vi "Main.vi"(11 "Module Admin":refnum<class "Delacor_lib_QMH_Module Admin.lvclass">) -> ()   [LabVIEW 2020, in "FileLogging.lvlib"]
doc: "This template is based off of the Queued Message Handler design pattern and the Queued Message Handler project template that ships with LabVIEW.\n\nThe main difference is that the queue is private to this module and communication between modules is performed via Broadcast and Request events.\n\nRequest events are wrapped in public API methods and are handled in the Event Handling Loop (EHL) of this VI. Any module can register for Broadcast events sent by this module. The EHL generates messages based on user interface actions.\n\nThe Message Handling Loop (MHL) processes messages generated by the EHL, or by other messages. The messages are string values, so new messages can be added easily to the Message Cases case structure in the MHL. Each message cluster can also provide an optional value for Message Data, which is a variant that can be converted to whatever message-specific data is required.\n_____\nBased on Delacor QMH Project Template 4.0.0.47.\n_____\nBased on Delacor QMH Project Template 5.0.0.82."
uses:
  FileLogging.lvlib
  <vilib>/Delacor/Delacor QMH/Libraries/Module Admin_class/Delacor_lib_QMH_Module Admin.lvclass
  Module Data--cluster.ctl
  Stop Argument--cluster.ctl
  <vilib>/Delacor/Delacor QMH/Libraries/Message Queue_class/Delacor_lib_QMH_Message Queue.lvclass/Delacor_lib_QMH_Message Queue.ctl
  <vilib>/Delacor/Delacor QMH/Libraries/Module Admin_class/Delacor_lib_QMH_Module Admin.lvclass/Delacor_lib_QMH_Module Admin.ctl
  Initialize File Argument--cluster.ctl
  Initialize File (Reply Payload)--cluster.ctl
  Log Data Argument--cluster.ctl
  Stop Logging Argument--cluster.ctl
  Settings Editor/Update Application Settings (Reply Payload)--cluster.ctl
  Settings Editor/Settings--cluster.ctl
  <vilib>/Utility/miscctls.llb/LVPointTypeDef.ctl
  <vilib>/Delacor/Delacor QMH/Libraries/Message Queue_class/Delacor_lib_QMH_Enqueue Message (Single).vi
  <vilib>/Delacor/Delacor QMH/Libraries/Module Admin_class/Delacor_lib_QMH_Get External Launch.vi
  <vilib>/Utility/error.llb/Error Cluster From Error Code.vi
  <vilib>/ErrorRing/Error Ring.xnode
  <vilib>/Delacor/Delacor QMH/Libraries/Message Queue_class/Delacor_lib_QMH_Message Queue.lvclass
  Settings Editor/Settings Editor.lvlib
panel:
  out "Settings":T1
  out "error out":errorcluster
  # "This is a headless module. Show its panel to confirm that the Settings are updated correctly and other debugging tasks. Use the Settings Editor to change the settings for this module."
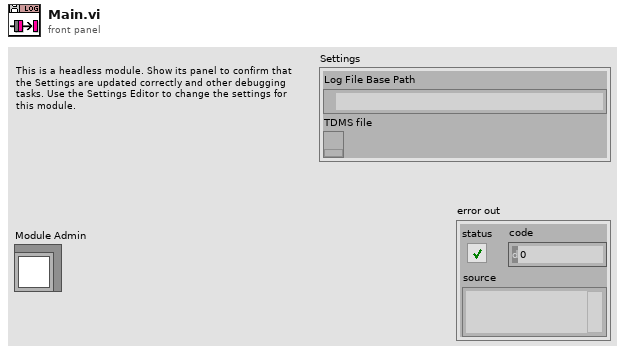
[diagram p1: front panel]
types:
  T1 = typedef "FileLogging.lvlib/Module Data--cluster.ctl" = cluster{"Log File Base Path":path, "TDMS file":refnum<k34>}
  T2 = typedef "Settings Editor.lvlib/Broadcast Events--cluster.ctl" = cluster{"Module Did Init":refnum<user-event>, "Status Updated":refnum<user-event>, "Error Reported":refnum<user-event>, "Module Did Stop":refnum<user-event>, "Update Module Execution Status":refnum<user-event>, "Application Settings Updated":refnum<user-event>}
  T3 = typedef "FileLogging.lvlib/Request Events--cluster.ctl" = cluster{"Stop Module":refnum<user-event>, "Show Panel":refnum<user-event>, "Hide Panel":refnum<user-event>, "Get Module Execution Status":refnum<user-event>, "Show Diagram":refnum<user-event>, "Stop Logging":refnum<user-event>, "Log Data":refnum<user-event>, "Initialize File":refnum<user-event>}
  T4 = enum32{"invalid lock state", "Not Locked", "Locked (No Password)", "Password-protected"}
  T5 = typedef "FileLogging.lvlib/Stop Argument--cluster.ctl" = cluster{"Origin":string, "Exit via Stop Module Req?":bool, "Wait for Module to stop?":bool}
  T6 = typedef "FileLogging.lvlib/Initialize File Argument--cluster.ctl" = cluster{"Wait Notifier":refnum<notifier>, "wait for reply":bool}
  T7 = typedef "FileLogging.lvlib/Log Data Argument--cluster.ctl" = cluster{"Waveforms":waveform(dbl)[]}
  T8 = typedef "FileLogging.lvlib/Stop Logging Argument--cluster.ctl" = cluster{"Boolean":bool}
  T9 = typedef "Settings Editor.lvlib/Update Application Settings (Reply Payload)--cluster.ctl" = cluster{"Settings":T10, "Update Settings_error":errorcluster}
  T10 = typedef "Settings Editor.lvlib/Settings--cluster.ctl" = cluster{"Log File Base Path":path, "Analog Input Channel":refnum<k21>, "Units":i32}
  T11 = typedef "LVPointTypeDef.ctl" = cluster{"Horizontal":i16, "Vertical":i16}
  T12 = enum32{"Invalid", "Standard", "Closed", "Hidden", "Minimized", "Maximized"}
  T13 = typedef "FileLogging.lvlib/Initialize File (Reply Payload)--cluster.ctl" = cluster{"File Path":path, "Initialize File_error":errorcluster}
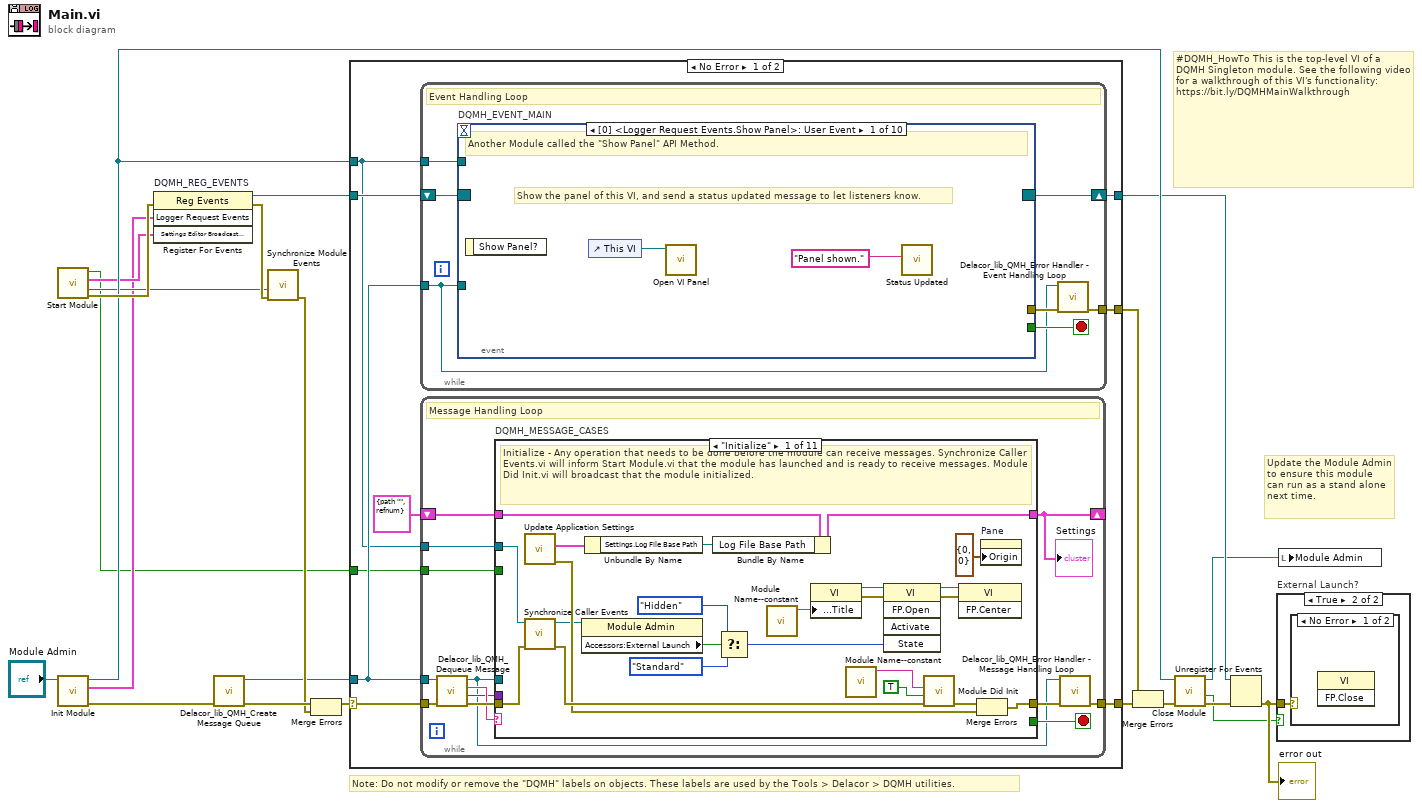
[diagram p0: block diagram]
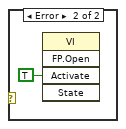
[diagram p3: hidden frame]
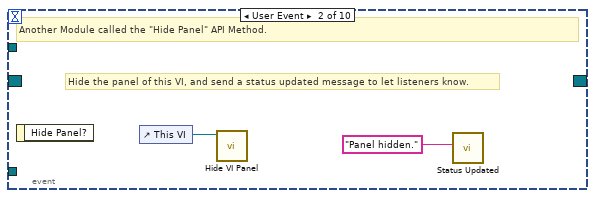
[diagram p4: hidden frame]
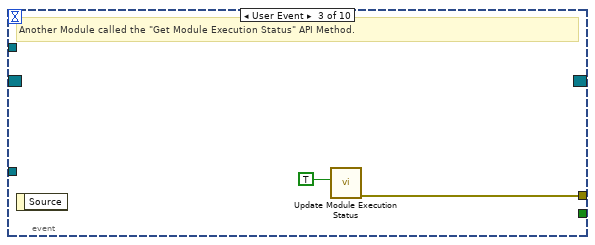
[diagram p5: hidden frame]
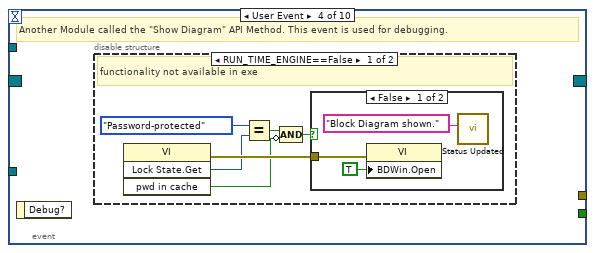
[diagram p6: hidden frame]
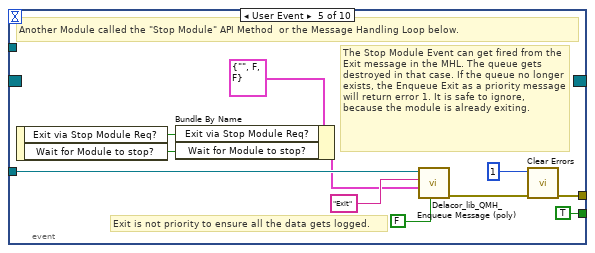
[diagram p9: hidden frame]
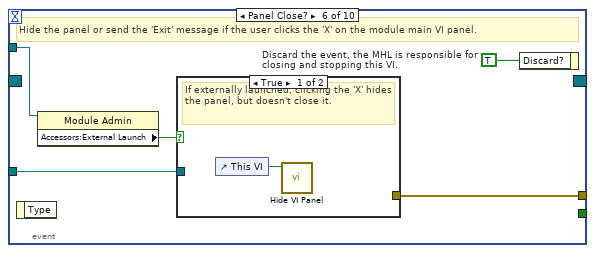
[diagram p10: hidden frame]
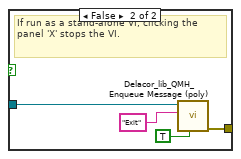
[diagram p11: hidden frame]
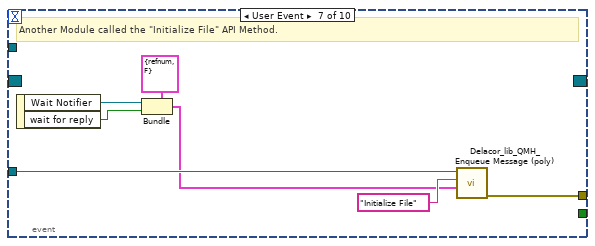
[diagram p12: hidden frame]
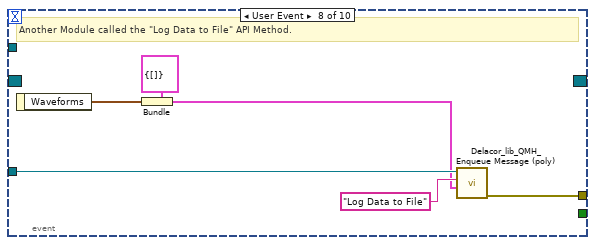
[diagram p13: hidden frame]
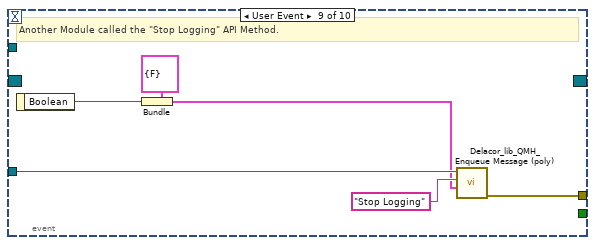
[diagram p14: hidden frame]
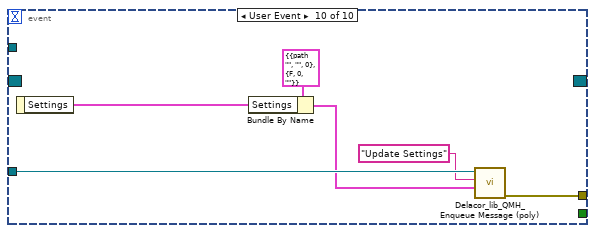
[diagram p15: hidden frame]
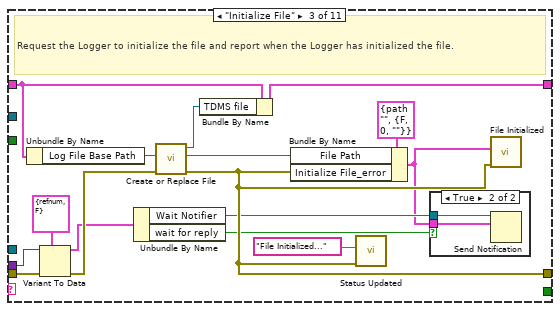
[diagram p17: hidden frame]
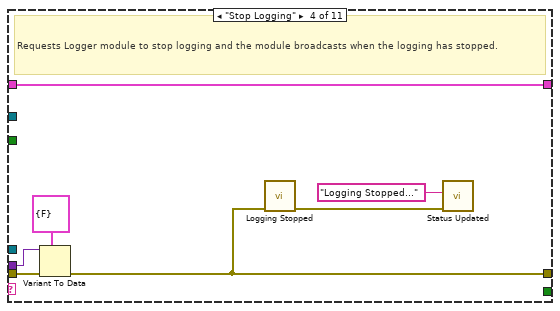
[diagram p19: hidden frame]
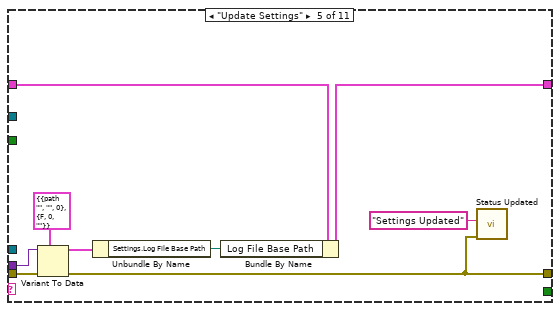
[diagram p20: hidden frame]
diagram:
  # "#DQMH_HowTo This is the top-level VI of a DQMH Singleton module. See the following video for a walkthrough of this VI's functionality: https://bit.ly/DQMHMainWalkthrough"
  # "Note: Do not modify or remove the \"DQMH\" labels on objects. These labels are used by the Tools > Delacor > DQMH utilities."
  # "Update the Module Admin to ensure this module can run as a stand alone next time."
  n1 = call "Start Module.vi"() -> ("error out"=w14:errorcluster, "Wait for Event Sync?"=w4:bool, "Settings Editor Broadcast Events"=w3:T2, "Module Was Already Running?"=w1:bool)  [unwired: 8 in]
  n2 = call "Init Module.vi"("Singleton Module Admin in"="Module Admin") -> ("error out"=w21:errorcluster, "Logger Request Events"=w2:T3, "Singleton Module Admin out"=w11:refnum<class "Delacor_lib_QMH_Module Admin.lvclass">)  [unwired: 8 in]
  n3 = register-events "DQMH_REG_EVENTS"(error in=w14, w2, w3) -> (reference out=w9:refnum<event-registration>, error out=w13:errorcluster)  [unwired: 1 in]
  n4 = call <vilib>:"Delacor_lib_QMH_Create Message Queue.vi"("error in (no error)"=w21) -> ("error out"=w16:errorcluster, "Message Queue"=w8:refnum<class "Delacor_lib_QMH_Message Queue.lvclass">)  [unwired: 9 in]
  n5 = call "Synchronize Module Events.vi"("error in (no error)"=w13, "Wait for Event Sync?"=w4) -> ("error out"=w12:errorcluster)  [unwired: 9 in]
  n6 = Merge Errors(w16, w12) -> (w15:errorcluster)
  n7 = case shown="No Error" w15 {
    selector: w15 -> [w29 w237]
    tunnel: [w31 w236] -> w22
    tunnel: [w28 w244] -> w10
    tunnel: w9 -> [w26 w244]
    tunnel: w8 -> [w25 w238]
    tunnel: [w30 _] -> w19
    tunnel: w11 -> [w24 w240]
    tunnel: w1 -> [w23 w239]
    frame No Error {
      n8 = while {
        tunnel: w25 -> [w32]
        shift-right: [w35] -> w28
        shift-left: w26 -> [w36]
        tunnel: [w37] -> w30
        tunnel: w24 -> [w33]
        stop <- w34 stop-if-true
        # "Event Handling Loop"
        n9 = event "DQMH_EVENT_MAIN" shown="[0] <Logger Request Events.Show Panel>: User Event" {
          selector: w36 -> [_ _ _ _ _ _ _ _ _ _]
          dyn-events: [_ _ _ _ _ _ _ _ _ _] -> w35
          timeout: _ -> [_ _ _ _ _ _ _ _ _ _]
          tunnel: [_ _ _ _ TRUE ("Discard?") _ _ _ _ _] -> w34
          tunnel: w32 -> [_ _ _ _ w60 w67 w80 w86 w92 w98]
          tunnel: [_ _ w44 _ w63 w69 w81 w87 w93 w99] -> w38
          tunnel: w33 -> [_ _ _ _ _ w66 _ _ _ _]
          event User Event {
            # "Show the panel of this VI, and send a status updated message to let listeners know."
            # "Another Module called the \"Show Panel\" API Method."
            n10 = event-data() -> ()  [unwired: 1 in, 1 out]
            n11 = control-ref of="This VI"() -> (w40:refnum<vi>)
            n12 = call "Open VI Panel.vi"("VI"=w40) -> ()  [unwired: 10 in, 1 out]
            n13 = call "Status Updated.vi"("Status"="Panel shown." ("format string")) -> ()  [unwired: 10 in, 1 out]
          }
          event User Event {
            # "Hide the panel of this VI, and send a status updated message to let listeners know."
            # "Another Module called the \"Hide Panel\" API Method."
            n14 = event-data() -> ()  [unwired: 1 in, 1 out]
            n15 = control-ref of="This VI"() -> (w42:refnum<vi>)
            n16 = call "Hide VI Panel.vi"("VI"=w42) -> ()  [unwired: 10 in, 1 out]
            n17 = call "Status Updated.vi"("Status"="Panel hidden." ("format string")) -> ()  [unwired: 10 in, 1 out]
          }
          event User Event {
            # "Another Module called the \"Get Module Execution Status\" API Method."
            n18 = event-data() -> ()  [unwired: 1 in, 1 out]
            n19 = call "Update Module Execution Status.vi"("Running?"=TRUE) -> ("error out"=w44:errorcluster)  [unwired: 10 in]
          }
          event User Event {
            # "Another Module called the \"Show Diagram\" API Method. This event is used for debugging."
            n20 = event-data() -> ()  [unwired: 1 in, 1 out]
            n21 = disable-structure shown="RUN_TIME_ENGINE==False" {
              frame condition #0 (active) {
                # "functionality not available in exe"
                n22 = invoke class="VI" method="Lock State.Get"() -> (error out=w50:errorcluster, "Get Lock State"=w49:T4, "pwd in cache"=w46:bool)  [unwired: 4 in, 1 out]
                n23 = Equal?(x=T4."Password-protected", y=w49) -> (x = y?=w47:bool)
                n24 = Compound Arithmetic op=AND(w47, invert w46) -> (w45:bool)
                n25 = case shown="False" w45 {
                  tunnel: w50 -> [w53 _]
                  frame False {
                    n26 = property class="VI"(error in=w53, "BDWin.Open"=TRUE ("Block Diagram Window:Open")) -> ()  [unwired: 1 in, 2 out]
                    n27 = call "Status Updated.vi"("Status"="Block Diagram shown." ("format string")) -> ()  [unwired: 10 in, 1 out]
                  }
                  frame True {
                    # "Password-protected VI, and the password is not in the cache. Do not show the diagram."
                  }
                }
              }
              frame condition #1 {
              }
            }
          }
          event User Event {
            # "Exit is not priority to ensure all the data gets logged."
            # "The Stop Module Event can get fired from the Exit message in the MHL. The queue gets destroyed in that case. If the queue no longer exists, the Enqueue Exit as a priority message will return error 1. It is safe to ignore, because the module is already exiting."
            # "Another Module called the \"Stop Module\" API Method  or the Message Handling Loop below."
            n28 = event-data() -> ("Exit via Stop Module Req?"=w56:bool, "Wait for Module to stop?"=w55:bool)  [unwired: 1 in]
            n29 = Bundle By Name(cluster=T5 {"Origin"="", "Exit via Stop Module Req?"=FALSE, "Wait for Module to stop?"=FALSE} ("Stop Argument"), "Exit via Stop Module Req?"=w56, "Wait for Module to stop?"=w55) -> (w54:T5)
            n30 = call-poly <vilib>:"Delacor_lib_QMH_Enqueue Message (poly).vi"("Priority Message? (F)"=FALSE, "Message Data"=w54, "Message"="Exit", "Message Queue in"=w60) -> ("error out"=w64:errorcluster)  [unwired: 6 in, 1 out]
            n31 = call <vilib>:"Clear Errors.vi"("error in (no error)"=w64, "specific error code to clear (0: all)"=1) -> ("error out"=w63:errorcluster)  [unwired: 4 in, 1 out]
          }
          event Panel Close? {
            w68 = TRUE  # Discard the event, the MHL is responsible for closing and stopping this VI.
            # "Hide the panel or send the 'Exit' message if the user clicks the 'X' on the module main VI panel."
            n32 = event-data() -> ()  [unwired: 1 in, 1 out]
            n33 = property class="Module Admin"(reference=w66) -> ("Accessors:External Launch"=w65:bool)  [unwired: 1 in, 2 out]
            n34 = case shown="True" w65 {
              tunnel: w67 -> [_ w73]
              tunnel: [_ w74] -> w69
              frame True {
                # "If externally launched, clicking the 'X' hides the panel, but doesn't close it."
                n35 = control-ref of="This VI"() -> (w70:refnum<vi>)
                n36 = call "Hide VI Panel.vi"("VI"=w70) -> ()  [unwired: 10 in, 1 out]
              }
              frame False {
                # "If run as a stand-alone VI, clicking the panel 'X' stops the VI."
                n37 = call-poly <vilib>:"Delacor_lib_QMH_Enqueue Message (poly).vi"("Priority Message? (F)"=TRUE, "Message"="Exit", "Message Queue in"=w73) -> ("error out"=w74:errorcluster)  [unwired: 7 in, 1 out]
              }
            }
            n38 = event-data("Discard?"=w68) -> ()  [unwired: 1 in, 1 out]
          }
          event User Event {
            # "Another Module called the \"Initialize File\" API Method."
            n39 = event-data() -> ("Wait Notifier"=w76:refnum<notifier>, "wait for reply"=w75:bool)  [unwired: 1 in]
            n40 = Bundle(cluster=T6 {"Wait Notifier"=refnum, "wait for reply"=FALSE} ("Initialize File Argument"), "Wait Notifier"=w76, "wait for reply"=w75) -> (w77:T6)
            n41 = call-poly <vilib>:"Delacor_lib_QMH_Enqueue Message (poly).vi"("Message Data"=w77, "Message"="Initialize File", "Message Queue in"=w80) -> ("error out"=w81:errorcluster)  [unwired: 7 in, 1 out]
          }
          event User Event {
            # "Another Module called the \"Log Data to File\" API Method."
            n42 = event-data() -> ("Waveforms"=w82:waveform(dbl)[])  [unwired: 1 in]
            n43 = Bundle(cluster=T7 {"Waveforms"=[]} ("Log Data to File Argument"), "Waveforms"=w82) -> (w83:T7)
            n44 = call-poly <vilib>:"Delacor_lib_QMH_Enqueue Message (poly).vi"("Message Data"=w83, "Message"="Log Data to File", "Message Queue in"=w86) -> ("error out"=w87:errorcluster)  [unwired: 7 in, 1 out]
          }
          event User Event {
            # "Another Module called the \"Stop Logging\" API Method."
            n45 = event-data() -> ("Boolean"=w88:bool)  [unwired: 1 in]
            n46 = Bundle(cluster=T8 {"Boolean"=FALSE} ("Stop Logging Argument"), "Boolean"=w88) -> (w89:T8)
            n47 = call-poly <vilib>:"Delacor_lib_QMH_Enqueue Message (poly).vi"("Message Data"=w89, "Message"="Stop Logging", "Message Queue in"=w92) -> ("error out"=w93:errorcluster)  [unwired: 7 in, 1 out]
          }
          event User Event {
            n48 = event-data() -> ("Settings"=w95:T10)  [unwired: 1 in]
            n49 = Bundle By Name(cluster=T9 {"Settings"={"Log File Base Path"=path "", "Analog Input Channel"="", "Units"=0}, "Update Settings_error"={"status"=FALSE, "code"=0, "source"=""}} ("Settings Updated Argument"), "Settings"=w95) -> (w94:T9)
            n50 = call-poly <vilib>:"Delacor_lib_QMH_Enqueue Message (poly).vi"("Message Data"=w94, "Message"="Update Settings", "Message Queue in"=w98) -> ("error out"=w99:errorcluster)  [unwired: 7 in, 1 out]
          }
        }
        n51 = call-dynamic "Delacor_lib_QMH_Error Handler - Event Handling Loop.vi"("error in (no error)"=w38, "Message Queue in"=w32) -> ("dup error in"=w37:errorcluster)  [unwired: 8 in, 1 out]
      }
      n52 = while {
        tunnel: w25 -> [w103]
        shift-right: [w107] -> _
        shift-left: T1 {"Log File Base Path"=path "", "TDMS file"=refnum} ("Data Cluster") -> [w108]
        tunnel: w29 -> [w111]
        tunnel: [w109] -> w31
        tunnel: w24 -> [w101]
        tunnel: w23 -> [w100]
        stop <- w106 stop-if-true
        # "Message Handling Loop"
        n53 = call-dynamic "Delacor_lib_QMH_Dequeue Message.vi"("error in (no error)"=w111, "Message Queue in"=w103) -> ("error out"=w110:errorcluster, "Message Data"=w104:variant, "Message"=w105:string, "Message Queue out"=w102:refnum<class "Delacor_lib_QMH_Message Queue.lvclass">)  [unwired: 6 in]
        n54 = case "DQMH_MESSAGE_CASES" shown="\"Initialize\"" w105 {
          selector: w105 -> [_ _ _ _ _ _ _ _ _ _ w223]
          tunnel: w102 -> [_ _ _ _ _ _ _ _ w189 w213 _]
          tunnel: w110 -> [w133 w137 w152 w162 w171 w180 w183 w185 w196 w219 w225]
          tunnel: [w130 w137 w153 w161 w164 w178 w182 w185 w192 w216 w226] -> w112
          tunnel: w108 -> [w120 w136 w141 w157 w170 w173 w181 w184 w191 w205 w224]
          tunnel: [w114 w136 w140 w157 w168 w173 w181 w184 w191 w205 w224] -> w107
          tunnel: [_ _ _ _ _ _ _ _ _ w212 _] -> w106
          tunnel: w104 -> [_ _ w150 w159 w169 w177 _ _ w190 w211 _]
          tunnel: w101 -> [w121 _ _ _ _ _ _ _ w188 w206 _]
          tunnel: w100 -> [_ _ _ _ _ _ _ _ _ w203 _]
          frame "Initialize" {
            # "Initialize - Any operation that needs to be done before the module can receive messages. Synchronize Caller Events.vi will inform Start Module.vi that the module has launched and is ready to receive messages. Module Did Init.vi will broadcast that the module initialized."
            n55 = call "Update Application Settings.vi"() -> ("error out"=w129:errorcluster, "Reply Payload"=w115:T9)  [unwired: 9 in, 1 out]
            n56 = call "Synchronize Caller Events.vi"("error in (no error)"=w133, "Singleton Module Admin in"=w121) -> ("error out"=w132:errorcluster, "Singleton Module Admin out"=w117:refnum<class "Delacor_lib_QMH_Module Admin.lvclass">)  [unwired: 8 in]
            n57 = property class="Module Admin"(reference=w117) -> ("Accessors:External Launch"=w125:bool)  [unwired: 1 in, 2 out]
            n58 = Unbundle By Name(w115) -> ("Settings.Log File Base Path"=w113:path)
            n59 = Bundle By Name(cluster=w120, "Log File Base Path"=w113) -> (w114:T1)
            n60 = Select(t=T12."Hidden" ("State"), s=w125, f=T12."Standard" ("State")) -> (s? t:f=w122:T12)
            n61 = call "Module Name--constant.vi"() -> ("Module Name"=w128:string)  [unwired: 11 in]
            n62 = property class="VI"("Front Panel.Title"=w128) -> (reference out=w127:refnum<vi>, error out=w135:errorcluster)  [unwired: 2 in]
            n63 = call "Module Name--constant.vi"() -> ("Module Name"=w118:string)  [unwired: 11 in]
            n64 = invoke class="VI" method="FP.Open"(reference=w127, error in=w135, "State"=w122) -> (reference out=w126:refnum<vi>, error out=w134:errorcluster)  [unwired: 2 in, 3 out]
            n65 = call "Module Did Init.vi"("error in (no error)"=w132, "Initialized?"=TRUE, "Origin"=w118) -> ("error out"=w131:errorcluster)  [unwired: 8 in]
            n66 = invoke class="VI" method="FP.Center"(reference=w126, error in=w134) -> ()  [unwired: 1 in, 3 out]
            n67 = Merge Errors(w131, w129) -> (w130:errorcluster)
            n68 = property on="Pane" class="Pane"("Origin"=T11 {"Horizontal"=0, "Vertical"=0}) -> ()  [unwired: 2 in, 2 out]
          }
          frame "--- Module Specific ---" {
            # "Separator -- The following cases handle messages specific to this Module."
          }
          frame "Initialize File" {
            # "Request the Logger to initialize the file and report when the Logger has initialized the file."
            n69 = Unbundle By Name(w141) -> ("Log File Base Path"=w143:path)
            n70 = Variant To Data(error in=w152, type=T6 {"Wait Notifier"=refnum, "wait for reply"=FALSE} ("Initialize File Argument"), Variant=w150) -> (data=w148:T6, error out=w151:errorcluster)
            n71 = Unbundle By Name(w148) -> ("Wait Notifier"=w147:refnum<notifier>, "wait for reply"=w146:bool)
            n72 = call "Create or Replace File.vi"("error in (no error)"=w151, "Log File Base Path"=w143) -> ("error out"=w153:errorcluster, "File Path"=w139:path, "Refnum out"=w142:refnum<k34>)  [unwired: 7 in]
            n73 = Bundle By Name(cluster=w141, "TDMS file"=w142) -> (w140:T1)
            n74 = Bundle By Name(cluster=T13 {"File Path"=path "", "Initialize File_error"={"status"=FALSE, "code"=0, "source"=""}} ("Initialize File (Reply Payload)"), "File Path"=w139, "Initialize File_error"=w153) -> (w144:T13)
            n75 = call "Status Updated.vi"("error in (no error)"=w153, "Status"="File Initialized...") -> ()  [unwired: 9 in, 1 out]
            n76 = case shown="True" w146 {
              tunnel: w147 -> [_ w155]
              tunnel: w144 -> [_ w154]
              frame False {
              }
              frame True {
                n77 = Send Notification(notification=w154, notifier=w155) -> ()  [unwired: 1 in, 2 out]
              }
            }
            n78 = call "File Initialized.vi"("error in (no error)"=w153, "Reply Payload"=w144) -> ()  [unwired: 9 in, 1 out]
          }
          frame "Stop Logging" {
            # "Requests Logger module to stop logging and the module broadcasts when the logging has stopped."
            n79 = Variant To Data(error in=w162, type=T8 {"Boolean"=FALSE} ("Stop Logging Argument"), Variant=w159) -> (error out=w161:errorcluster)  [unwired: 1 out]
            n80 = call "Logging Stopped.vi"("error in (no error)"=w161) -> ("error out"=w160:errorcluster)  [unwired: 10 in]
            n81 = call "Status Updated.vi"("error in (no error)"=w160, "Status"="Logging Stopped...") -> ()  [unwired: 9 in, 1 out]
          }
          frame "Update Settings" {
            n82 = Variant To Data(error in=w171, type=T9 {"Settings"={"Log File Base Path"=path "", "Analog Input Channel"="", "Units"=0}, "Update Settings_error"={"status"=FALSE, "code"=0, "source"=""}} ("Settings Updated Argument"), Variant=w169) -> (data=w167:T9, error out=w164:errorcluster)
            n83 = Unbundle By Name(w167) -> ("Settings.Log File Base Path"=w166:path)
            n84 = Bundle By Name(cluster=w170, "Log File Base Path"=w166) -> (w168:T1)
            n85 = call "Status Updated.vi"("error in (no error)"=w164, "Status"="Settings Updated") -> ()  [unwired: 9 in, 1 out]
          }
          frame "Log Data to File" {
            # "Requests Logger module to log data to file"
            n86 = Variant To Data(error in=w180, type=T7 {"Waveforms"=[]} ("Log Data to File Argument"), Variant=w177) -> (data=w175:T7, error out=w179:errorcluster)
            n87 = Unbundle By Name(w173) -> ("TDMS file"=w172:refnum<k34>)
            n88 = Unbundle By Name(w175) -> ("Waveforms"=w174:waveform(dbl)[])
            n89 = call "Log Data to File.vi"("error in (no error)"=w179, "Data to log"=w174, "TDMS File Reference"=w172) -> ("error out"=w178:errorcluster)  [unwired: 8 in]
          }
          frame "---Copy This Frame---" {
            # "Duplicate this frame when creating new messages.  Change this comment in the duplicated frame to describe this message."
            n90 = Merge Errors(w183) -> (w182:errorcluster)
          }
          frame "--- Exit and Error Handling---" {
            # "Separator - The following cases handle errors and exit messages."
          }
          frame "Error" {
            # "Error - Check the error message data and respond accordingly. This message is sent by the \"Error Handler\" VIs at the end of each loop in this application."
            n91 = property class="Module Admin"(reference=w188) -> ("Accessors:External Launch"=w187:bool)  [unwired: 1 in, 2 out]
            n92 = Variant To Data(error in=w196, type=errorcluster {"status"=FALSE, "code"=0, "source"=""} ("error constant"), Variant=w190) -> (data=w197:errorcluster, error out=w194:errorcluster)
            n93 = call "Module Name--constant.vi"() -> ("Module Name"=w186:string)  [unwired: 11 in]
            n94 = call "Error Reported.vi"("Additional Information"=w186, "Error"=w197) -> ()  [unwired: 9 in, 1 out]
            n95 = case shown="False" w187 {
              tunnel: [w202 _] -> w193
              tunnel: w189 -> [w200 _]
              tunnel: w197 -> [w201 _]
              frame False {
                # "If the module is running standalone, then pop up an error dialog and call the \"Exit\" message."
                n96 = call <vilib>:"Simple Error Handler.vi"("error in (no error)"=w201) -> ()  [unwired: 4 in, 5 out]
                n97 = call-poly <vilib>:"Delacor_lib_QMH_Enqueue Message (poly).vi"("Priority Message? (F)"=TRUE, "Message"="Exit", "Message Queue in"=w200) -> ("error out"=w202:errorcluster)  [unwired: 7 in, 1 out]
              }
              frame True {
                # "If the module was launched externally, calling the Error Reported broadcast VI is the only action performed by the \"Error\" message. The module's caller can then process the error appropriately."
              }
            }
            n98 = Merge Errors(w194, w193) -> (w192:errorcluster)
            n99 = local write "error out"(w192) -> ()
          }
          frame "Exit" {
            w210 = 91  # 91: not all Exit messages will have an argument
            w212 = TRUE  # Stop the VI
            # "Release the message queue reference"
            # "Exit - Exit the application."
            n100 = Variant To Data(error in=w219, type=T5 {"Origin"="", "Exit via Stop Module Req?"=FALSE, "Wait for Module to stop?"=FALSE} ("Stop Argument"), Variant=w211) -> (data=w208:T5, error out=w215:errorcluster)
            n101 = Unbundle By Name(w205) -> ("TDMS file"=w204:refnum<k34>)
            n102 = call <vilib>:"Clear Errors.vi"("error in (no error)"=w215, "specific error code to clear (0: all)"=w210) -> ("error out"=w218:errorcluster)  [unwired: 4 in, 1 out]
            n103 = control-ref of="This VI"() -> (w207:refnum<vi>)
            n104 = call-dynamic "Delacor_lib_QMH_Release Message Queue.vi"("error in (no error)"=w218, "Message Queue"=w213) -> ("error out"=w217:errorcluster)  [unwired: 9 in]
            n105 = call "Handle Exit.vi"("Stop Argument"=w208, "Admin in"=w206, "VI reference"=w207) -> ("error out"=w214:errorcluster)  [unwired: 7 in, 1 out]
            n106 = call "Close File.vi"("Refnum out"=w204) -> ()  [unwired: 10 in, 1 out]
            n107 = case "Settings Editor was\nalready running?" shown="False" w203 {
              frame False {
                n108 = call "Module Name--constant.vi"() -> ("Module Name"=w221:string)  [unwired: 11 in]
                n109 = call "Stop Module.vi"("Wait for Module to Stop? (F)"=TRUE, "Origin"=w221) -> ()  [unwired: 9 in, 1 out]
              }
              frame True {
                # "Another Module is\nin charge of stopping Settings Editor"
              }
            }
            n110 = Merge Errors(w217, w214) -> (w216:errorcluster)
          }
          frame Default {
            # "'Default' case only runs if there is a message that isn't defined in any of the other cases.  Output a programming error."
            n111 = call "Module Name--constant.vi"() -> ("Module Name"=w222:string)  [unwired: 11 in]
            n112 = xnode "Error Ring"("parameter 0"=w223, "parameter 1"=w222) -> ("error out"=w227:errorcluster)
            n113 = Merge Errors(w225, w227) -> (w226:errorcluster)
          }
        }
        "Settings" <- w107
        n114 = call-dynamic "Delacor_lib_QMH_Error Handler - Message Handling Loop.vi"("error in (no error)"=w112, "Message Queue in"=w102) -> ("dup error in"=w109:errorcluster)  [unwired: 8 in, 1 out]
      }
    }
    frame Error {
      # "Synchronize Caller Events.vi will inform Start Module.vi that the module has launched and will let the code calling Start Module.vi register for broadcasts and would permit the caller receive the broadcast that an error occurred at launch time."
      n115 = call "Synchronize Caller Events.vi"("Singleton Module Admin in"=w240) -> ("error out"=w245:errorcluster)  [unwired: 9 in, 1 out]
      n116 = call-dynamic "Delacor_lib_QMH_Release Message Queue.vi"("error in (no error)"=w237, "Message Queue"=w238) -> ("error out"=w236:errorcluster)  [unwired: 9 in]
      n117 = call "Module Name--constant.vi"() -> ("Module Name"=w243:string)  [unwired: 11 in]
      n118 = case "Settings Editor was\nalready running?" shown="False" w239 {
        frame False {
          n119 = call "Module Name--constant.vi"() -> ("Module Name"=w248:string)  [unwired: 11 in]
          n120 = call "Stop Module.vi"("Wait for Module to Stop? (F)"=TRUE, "Origin"=w248) -> ()  [unwired: 9 in, 1 out]
        }
        frame True {
          # "Another Module is\nin charge of stopping Settings Editor"
        }
      }
      n121 = Format Into String(format string="An error occurred during initialization. %s is no longer running.", w243) -> (resulting string=w241:string)  [unwired: 2 in, 1 out]
      n122 = Merge Errors(w237, w245) -> (w246:errorcluster)
      n123 = call "Error Reported.vi"("Additional Information"=w241, "Error"=w246) -> ()  [unwired: 9 in, 1 out]
    }
  }
  n124 = Merge Errors(w19, w22) -> (w18:errorcluster)
  n125 = call "Close Module.vi"("error in (no error)"=w18, "Module Admin in"=w11) -> ("error out"=w20:errorcluster, "External Launch"=w5:bool, "Module Admin out"=w6:refnum<class "Delacor_lib_QMH_Module Admin.lvclass">)  [unwired: 7 in]
  n126 = Unregister For Events(event registration refnum=w10, error in=w20) -> (error out=w17:errorcluster)
  "error out" <- w17
  n127 = case "External Launch?" shown="True" w5 {
    tunnel: w17 -> [_ w249]
    frame False {
    }
    frame True {
      n128 = case shown="No Error" w249 {
        frame No Error {
          n129 = invoke class="VI" method="FP.Close"() -> ()  [unwired: 3 in, 3 out]
        }
        frame Error {
          n130 = invoke class="VI" method="FP.Open"("Activate"=TRUE ("Activate?")) -> ()  [unwired: 4 in, 5 out]
        }
      }
    }
  }
  n131 = local write "Module Admin"(w6) -> ()
